vi "Display Data to Table.vi"(11 "Macro":T1) -> (1 "Metadata":string, 3 "Macro Steps":string[][](array[string]))   [LabVIEW 2023]
doc: "Converts <B>Macro</B> to a table of macro steps and a string of associated metadata."
uses:
  CTLs/Macro Cluster V3.ctl
  CTLs/Macro Config V3.ctl
  CTLs/Step V3.ctl
  CTLs/Step Type V3.ctl
panel:
  in  "Virtual Key":u8(ring)=65
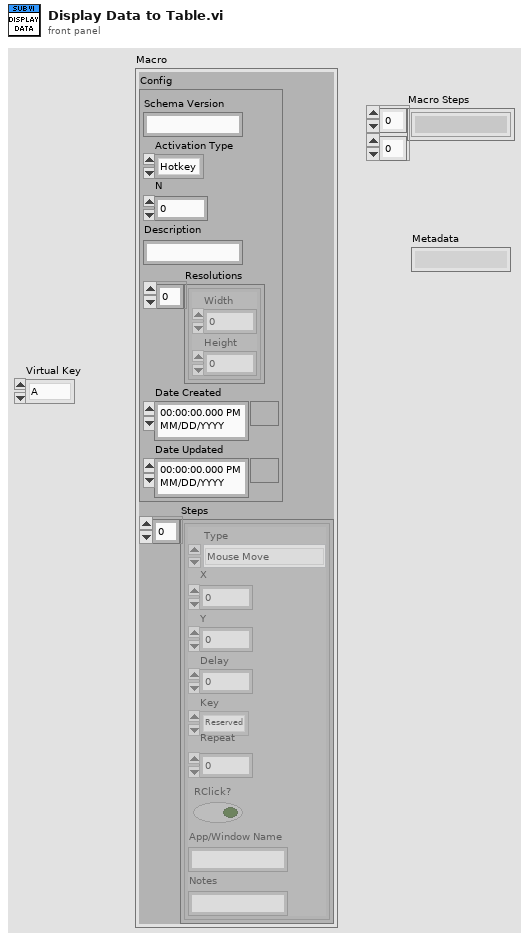
[diagram p1: front panel]
types:
  T1 = typedef "Macro Cluster V3.ctl" = cluster{"Config":T2, "Steps":T3[]}
  T2 = typedef "Macro Config V3.ctl" = cluster{"Schema Version":string, "Activation Type":enum32{"Hotkey", "Automatic"}, "N":i32, "Description":string, "Resolutions":cluster{"Width":i16, "Height":i16}[], "Date Created":timestamp, "Date Updated":timestamp}
  T3 = typedef "Step V3.ctl" = cluster{"Type":T4, "X":i32, "Y":i32, "Delay":i32, "Key":u8, "Repeat":i32, "RClick?":bool, "App/Window Name":string, "Notes":string}
  T4 = typedef "Step Type V3.ctl" = enum16{"Mouse Move", "Mouse Click", "Key Press", "Wait", "Mouse Down", "Mouse Up", "Key Down", "Key Up", "Run Application", "Maximize Window", "Restore Window", "Minimize Window", "Close Window", "Bring Window to Front", "Send Window to Back"}
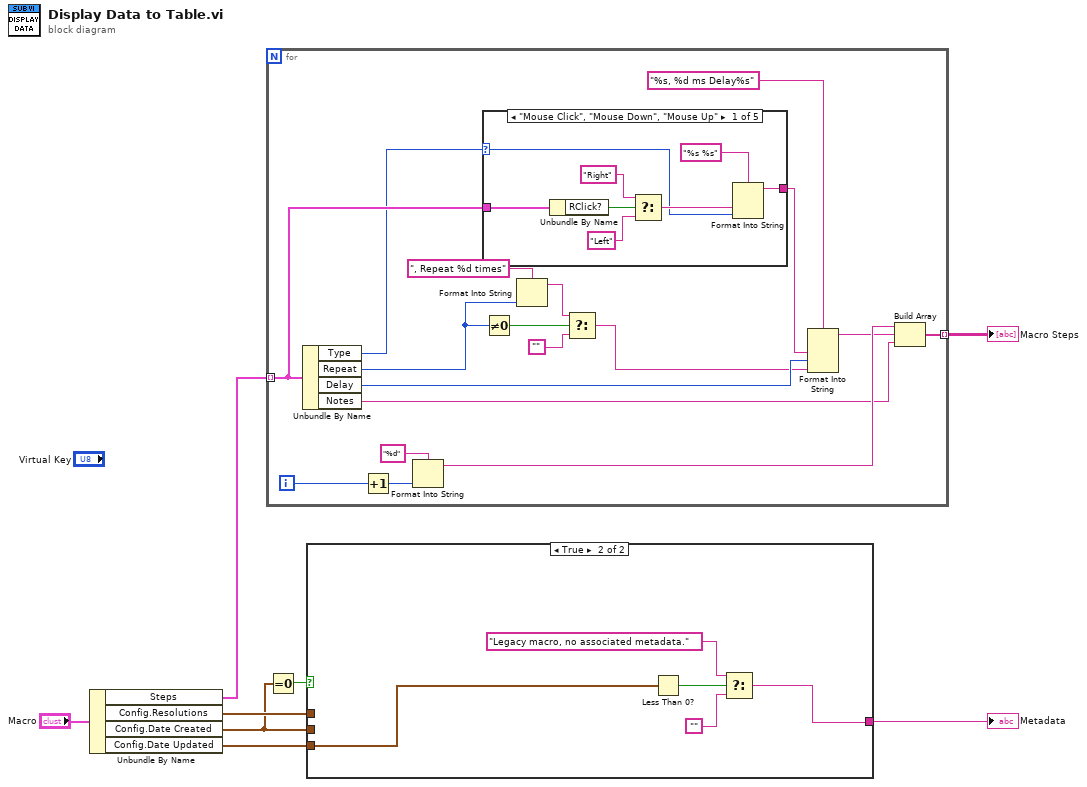
[diagram p0: block diagram]
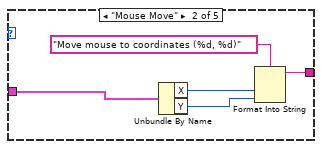
[diagram p2: hidden frame]
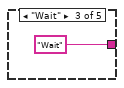
[diagram p3: hidden frame]
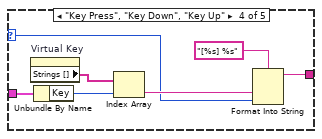
[diagram p4: hidden frame]
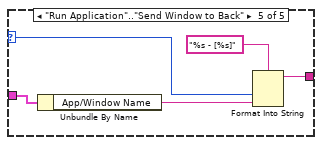
[diagram p5: hidden frame]
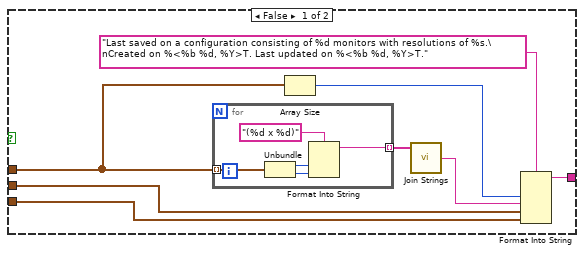
[diagram p6: hidden frame]
diagram:
  n1 = Unbundle By Name("Macro") -> ("Steps"=w6:T3[], "Config.Resolutions"=w4:cluster{"Width":i16, "Height":i16}[], "Config.Date Created"=w1:timestamp, "Config.Date Updated"=w5:timestamp)
  n2 = for {
    tunnel: w6 -> [w25] mode=indexing
    tunnel: [w20] -> w8 mode=indexing
    i -> [w22]
    n3 = Unbundle By Name(w25) -> ("Type"=w11:T4, "Repeat"=w17:i32, "Delay"=w19:i32, "Notes"=w9:string)
    n4 = Increment(x=w22) -> (x+1=w24:i32)
    n5 = Format Into String(format string="%d", w24) -> (resulting string=w21:string)  [unwired: 2 in, 1 out]
    n6 = case shown="\"Mouse Click\", \"Mouse Down\", \"Mouse Up\"" w11 {
      selector: w11 -> [w28 _ _ w42 w50]
      tunnel: w25 -> [w30 w39 _ w47 w52]
      tunnel: [w27 w38 "Wait" w41 w49] -> w12
      frame "Mouse Click", "Mouse Down", "Mouse Up" {
        n7 = Unbundle By Name(w30) -> ("RClick?"=w33:bool)
        n8 = Select(t="Right", s=w33, f="Left") -> (s? t:f=w29:string)
        n9 = Format Into String(format string="%s %s", w29, w28) -> (resulting string=w27:string)  [unwired: 2 in, 1 out]
      }
      frame "Mouse Move" {
        n10 = Unbundle By Name(w39) -> ("X"=w36:i32, "Y"=w35:i32)
        n11 = Format Into String(format string="Move mouse to coordinates (%d, %d)", w36, w35) -> (resulting string=w38:string)  [unwired: 2 in, 1 out]
      }
      frame "Wait" {
      }
      frame "Key Press", "Key Down", "Key Up" {
        n12 = property on="Virtual Key" class="Ring (strict)"() -> ("Strings []"=w45:string[])  [unwired: 2 in, 2 out]
        n13 = Unbundle By Name(w47) -> ("Key"=w44:u8)
        n14 = Index Array(array=w45, index=w44) -> (element=w43:string)
        n15 = Format Into String(format string="[%s] %s", w43, w42) -> (resulting string=w41:string)  [unwired: 2 in, 1 out]
      }
      frame "Run Application".."Send Window to Back" {
        n16 = Unbundle By Name(w52) -> ("App/Window Name"=w48:string)
        n17 = Format Into String(format string="%s - [%s]", w50, w48) -> (resulting string=w49:string)  [unwired: 2 in, 1 out]
      }
    }
    n18 = Not Equal To 0?(x=w17) -> (x != 0?=w16:bool)
    n19 = Format Into String(format string=", Repeat %d times", w17) -> (resulting string=w15:string)  [unwired: 2 in, 1 out]
    n20 = Select(t=w15, s=w16, f="") -> (s? t:f=w13:string)
    n21 = Format Into String(format string="%s, %d ms Delay%s", w12, w19, w13) -> (resulting string=w10:string)  [unwired: 2 in, 1 out]
    n22 = Build Array(w21, w10, w9) -> (w20:string[])
  }
  "Macro Steps" <- w8
  n23 = Equal To 0?(x=w1) -> (x = 0?=w2:bool)
  n24 = case shown="True" w2 {
    tunnel: w5 -> [w59 w70]
    tunnel: w1 -> [w58 _]
    tunnel: w4 -> [w56 _]
    tunnel: [w53 w66] -> w3
    frame False {
      n25 = for {
        tunnel: w56 -> [w64] mode=indexing
        tunnel: [w61] -> w55 mode=indexing
        n26 = Unbundle(w64) -> ("Width"=w62:i16, "Height"=w63:i16)
        n27 = Format Into String(format string="(%d x %d)", w62, w63) -> (resulting string=w61:string)  [unwired: 2 in, 1 out]
      }
      n28 = Array Size(array=w56) -> (size(s)=w57:i32)
      n29 = call <vilib>:"Join Strings.vi"("Strings In"=w55) -> ("String"=w54:string)  [unwired: 2 in]
      n30 = Format Into String(format string="Last saved on a configuration consisting of %d monitors with resolutions of %s.\nCreated on %<%b %d, %Y>T. Last updated on %<%b %d, %Y>T.", w57, w54, w58, w59) -> (resulting string=w53:string)  [unwired: 2 in, 1 out]
    }
    frame True {
      n31 = Less Than 0?(x=w70) -> (x < 0?=w69:bool)
      n32 = Select(t="Legacy macro, no associated metadata.", s=w69, f="") -> (s? t:f=w66:string)
    }
  }
  "Metadata" <- w3
